vi "Hall Effect Data.vi"() -> ()   [LabVIEW 2016, in "Hall Effect Library.lvlib"]
uses:
  Hall Effect Library.lvlib
panel:
  in  "8-Contact Sample Hall Results":cluster{"RH":dbl, "uH":dbl}
  in  "8-Contact Sample Hall Currents":dbl[](array[numeric])
  in  "8-Contact Sample Hall Voltages":dbl[](array[numeric])
  in  "6-Contact Sample Hall Results":T1
  in  "6-Contact Sample Hall Currents":dbl[](array[numeric])
  in  "6-Contact Sample Hall Voltages":dbl[](array[numeric])
  in  "8-Contact Sample Resistivity Results":cluster{"PAvg":dbl, "PA":dbl, "PB":dbl}
  in  "8-Contact Sample Resistivity Currents":dbl[](array[numeric])
  in  "8-Contact Sample Resistivity Voltages":dbl[](array[numeric])
  in  "6-Contact Sample Resistivity Results":cluster{"PAvg":dbl, "PA":dbl, "PB":dbl}
  in  "6-Contact Sample Resistivity Currents":dbl[](array[numeric])
  in  "6-Contact Sample Resistivity Voltages":dbl[](array[numeric])=[0.0, 0.0, 0.0, 0.0]
  in  "Bar Sample Hall Results":cluster{"n/p":dbl, "uH":dbl}
  in  "Bar Sample Hall Currents":dbl[](array[numeric])
  in  "Bar Sample Hall Voltages":dbl[](array[numeric])=[0.0]
  in  "Bar Sample Resistivity Results":cluster{"p":dbl}
  in  "Bar Sample Resistivity Currents":dbl[](array[numeric])
  in  "Bar Sample Resistivity Voltages":dbl[](array[numeric])
  in  "HE Currents":dbl[](array[numeric])=[0.0, 0.0, 0.0, 0.0, 0.0, 0.0, 0.0, 0.0]
  in  "VDP Currents":dbl[](array[numeric])=[0.0, 0.0, 0.0, 0.0, 0.0, 0.0, 0.0, 0.0]
  in  "HE Results":T2
  in  "VDP Results":T3
  in  "HE Voltages":dbl[](array[numeric])=[0.0, 0.0, 0.0, 0.0, 0.0, 0.0, 0.0, 0.0]
  in  "VDP Voltages":dbl[](array[numeric])=[0.0, 0.0, 0.0, 0.0, 0.0, 0.0, 0.0, 0.0]
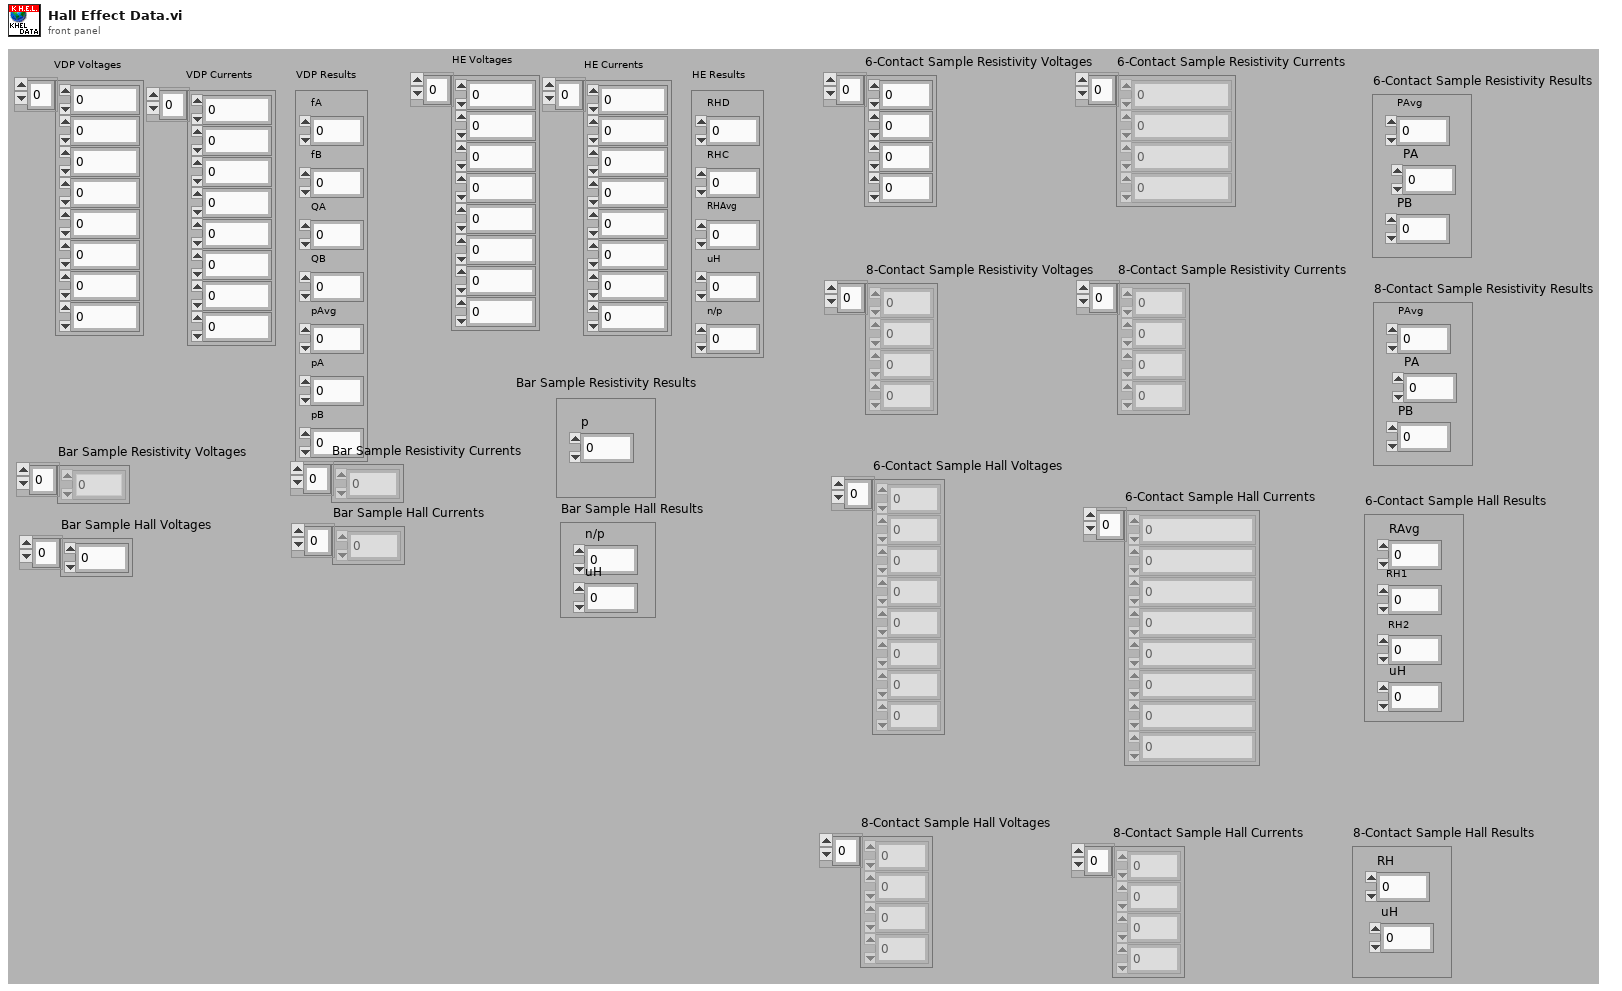
[diagram p1: front panel]
types:
  T1 = cluster{"RAvg":dbl, "RH1":dbl, "RH2":dbl, "uH":dbl}
  T2 = cluster{"RHD":dbl, "RHC":dbl, "RHAvg":dbl, "uH":dbl, "n/p":dbl}
  T3 = cluster{"fA":dbl, "fB":dbl, "QA":dbl, "QB":dbl, "pAvg":dbl, "pA":dbl, "pB":dbl}
diagram:
